vi "Digital Read 1 Channel.vi"(8 "error in (no error)":errorcluster, 10 "Channel":i32, 11 "NI-DAQ in":refnum<class "NI-DAQ.lvclass">) -> (0 "error out":errorcluster, 2 "Value":bool=TRUE, 3 "NI-DAQ out":refnum<class "NI-DAQ.lvclass">)   [LabVIEW 2020, in "NI-DAQ.lvclass"]
uses:
  NI-DAQ.lvclass
panel:
  out "index":i32
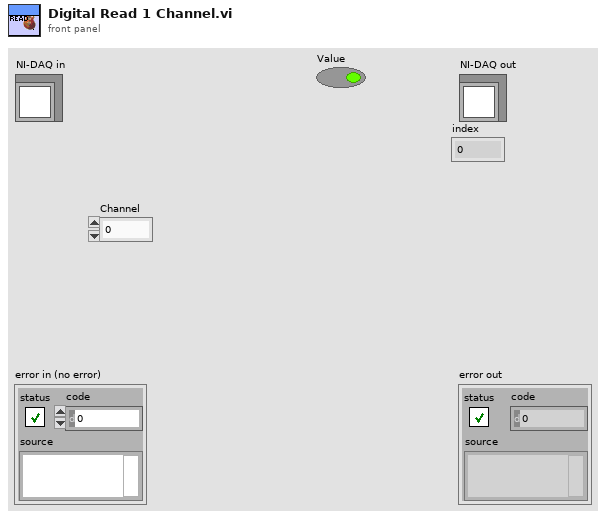
[diagram p1: front panel]
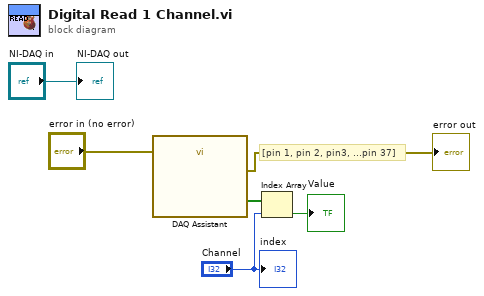
[diagram p0: block diagram]
diagram:
  # "[pin 1, pin 2, pin3, ...pin 37]"
  n1 = call "DAQ Assistant"("error in"="error in (no error)") -> ("data"=w2:bool[], "error out"=→"error out":errorcluster)  [unwired: 16 in, 1 out]
  n2 = Index Array(array=w2, index="Channel") -> (element=→"Value":bool)
  "NI-DAQ out" <- "NI-DAQ in"
  "index" <- "Channel"
